vi "validate student data.vi"(6 "periods per day":i32, 9 "Student data":i32[][](array[numeric]), 11 "course periods":i32[](array[numeric])) -> (1 "validated Student data":i32[][](array[numeric]))   [LabVIEW 2009]
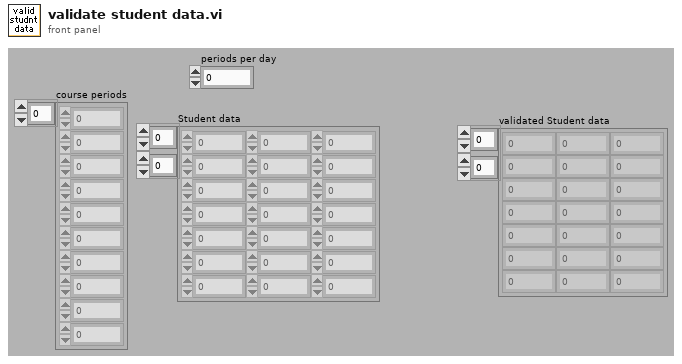
[diagram p1: front panel]
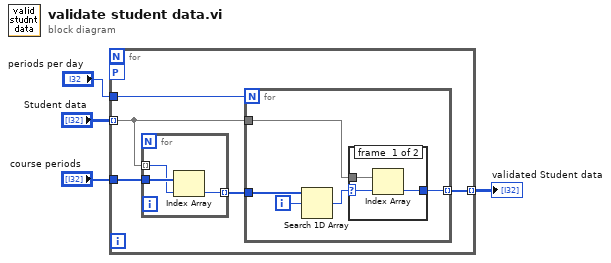
[diagram p0: block diagram]
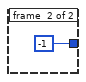
[diagram p2: hidden frame]
diagram:
  n1 = for {
    tunnel: "Student data" -> [w6] mode=indexing
    tunnel: "course periods" -> [w9]
    tunnel: [w7] -> w2 mode=indexing
    tunnel: "periods per day" -> [w5]
    workers-P: _ -> [_]
    n2 = for {
      tunnel: w6 -> [w20] mode=indexing
      tunnel: w9 -> [w21]
      tunnel: [w19] -> w8 mode=indexing
      n3 = Index Array(array=w21, index=w20) -> (element=w19:i32)
    }
    n4 = for {
      N: w5 -> [_]
      tunnel: w8 -> [w14]
      tunnel: w6 -> [w11]
      tunnel: [w10] -> w7 mode=indexing
      i -> [w13]
      n5 = Search 1D Array(1D array=w14, element=w13) -> (index of element=w12:i32)  [unwired: 1 in]
      n6 = case shown="-1" w12 {
        selector: w12 -> [w17 _]
        tunnel: w11 -> [w16 _]
        tunnel: [w15 -1 ("class course ID")] -> w10
        frame #0 {
          n7 = Index Array(array=w16, index=w17) -> (element=w15:i32)
        }
        frame #1 {
        }
      }
    }
  }
  "validated Student data" <- w2
